vi "Read_MultiplexerBuffer.vi"(8 "error in (no error)":errorcluster, 11 "Multiplexer_Opmux in":refnum<class "Multiplexer_Opmux.lvclass">) -> (0 "error out":errorcluster, 2 "BufferOut":string, 3 "Multiplexer_Opmux out":refnum<class "Multiplexer_Opmux.lvclass">)   [LabVIEW 2013, in "Multiplexer_Opmux.lvclass"]
uses:
  Multiplexer_Opmux.lvclass
  Multiplexer_Opmux.lvclass/Multiplexer_Opmux.ctl
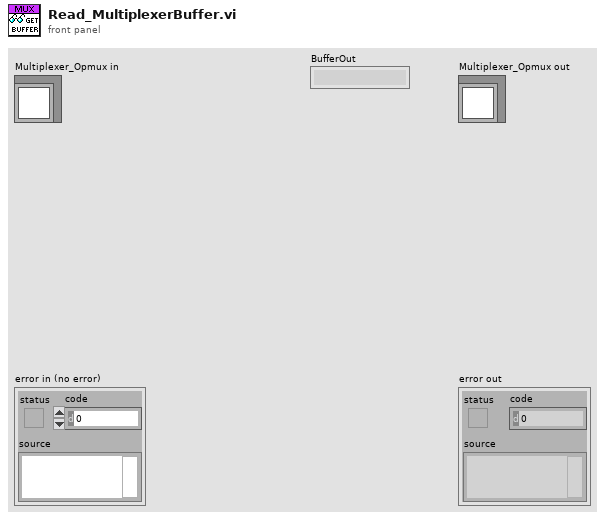
[diagram p1: front panel]
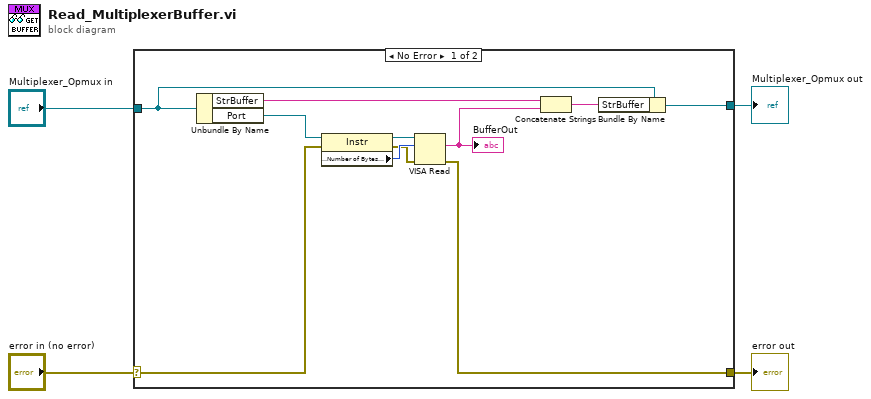
[diagram p0: block diagram]
diagram:
  n1 = case shown="No Error" "error in (no error)" {
    selector: "error in (no error)" -> [w12 w17]
    tunnel: [w10 w17] -> w3
    tunnel: [w9 w16] -> w1
    tunnel: "Multiplexer_Opmux in" -> [w5 w16]
    frame No Error {
      n2 = Unbundle By Name(w5) -> ("StrBuffer"=w7:string, "Port"=w15:refnum<visa-resource-name>)
      n3 = property class="Instr"(reference=w15, error in=w12) -> (reference out=w14:refnum<visa-resource-name>, error out=w11:errorcluster, "Serial Settings:Number of Bytes at Serial Port"=w13:u32)
      n4 = VISA Read(VISA resource name=w14, byte count=w13, error in (no error)=w11) -> (read buffer=w6:string, error out=w10:errorcluster)  [unwired: 2 out]
      "BufferOut" <- w6
      n5 = Concatenate Strings(w7, w6) -> (w8:string)
      n6 = Bundle By Name(cluster=w5, "StrBuffer"=w8) -> (w9:refnum<class "Multiplexer_Opmux.lvclass">)
    }
    frame Error {
    }
  }
  "error out" <- w3
  "Multiplexer_Opmux out" <- w1
